vi "XY Drift Test.vi"() -> ()   [LabVIEW 2016]
panel:
  in  "Frame Trigger":i32=500
  out "Frame Number":i32
  out "error out":errorcluster
  in  "Auto XY":bool=TRUE
  out "XY On":bool
  in  "Quit":bool
  in  "Set True":bool
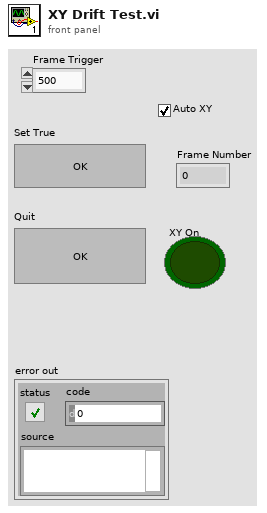
[diagram p1: front panel]
types:
  T1 = typedef "Image Type" = u32
  T2 = typedef "IMAQ Image.ctl" = refnum<image>
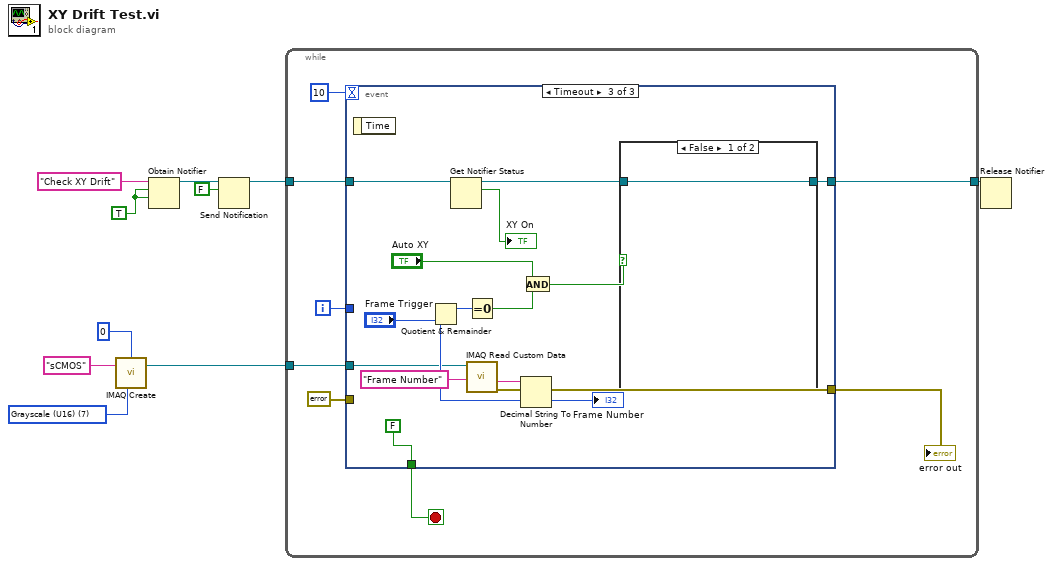
[diagram p0: block diagram]
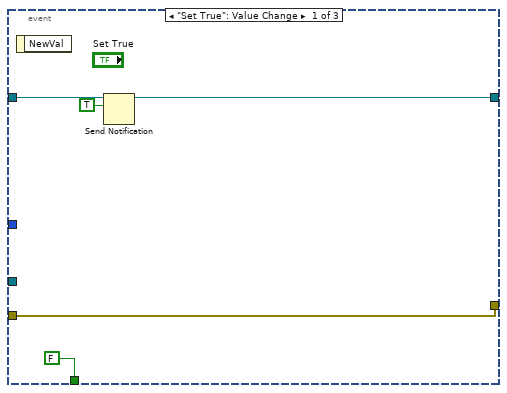
[diagram p2: hidden frame]
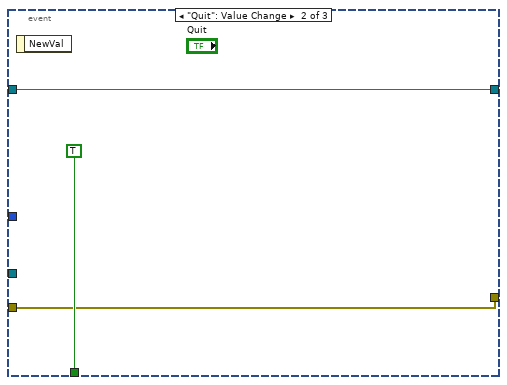
[diagram p3: hidden frame]
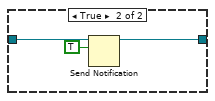
[diagram p4: hidden frame]
diagram:
  w2 = T1 7 items=["Grayscale (U8)", "Grayscale (I16)", "Grayscale (SGL)", "Complex (CSG)", "RGB (U32)", "HSL (U32)", "RGB (U64)", "Grayscale (U16)"] ("Image Type")
  w10 = TRUE ("create if not found? (T)")
  n1 = call "IMAQ Create"("Border Size"=0, "Image Name"="sCMOS" ("name (unnamed)"), "Image Type"=w2) -> ("New Image"=w4:T2)  [unwired: 2 in, 1 out]
  n2 = Obtain Notifier(name (unnamed)="Check XY Drift", notification data type=w10, create if not found? (T)=w10) -> (notifier out=w8:refnum<notifier>)  [unwired: 1 in, 2 out]
  n3 = Send Notification(notification=FALSE, notifier=w8) -> (notifier out=w6:refnum<notifier>)  [unwired: 1 in, 1 out]
  n4 = while {
    tunnel: w6 -> [w17]
    tunnel: [w16] -> w5
    tunnel: w4 -> [w11]
    i -> [w15]
    stop <- w18 stop-if-true
    n5 = event shown="[2] Timeout" {
      selector: _ -> [_ _ _]
      dyn-events: _ -> [_ _ _]
      timeout: 10 -> [_ _ _]
      tunnel: [FALSE ("notification") TRUE ("notification") FALSE ("notification")] -> w18
      tunnel: w17 -> [w22 w26 w40]
      tunnel: [w21 w26 w36] -> w16
      tunnel: w15 -> [_ _ _]
      tunnel: [w19 w24 w31] -> w13
      tunnel: errorcluster {"status"=FALSE, "code"=0, "source"=""} ("error in (no error)") -> [w19 w24 _]
      tunnel: w11 -> [_ _ w29]
      event "Set True": Value Change {
        n6 = event-data() -> ()  [unwired: 1 in, 1 out]
        n7 = Send Notification(notification=TRUE, notifier=w22) -> (notifier out=w21:refnum<notifier>)  [unwired: 1 in, 1 out]
      }
      event "Quit": Value Change {
        n8 = event-data() -> ()  [unwired: 1 in, 1 out]
      }
      event Timeout {
        n9 = event-data() -> ()  [unwired: 1 in, 1 out]
        n10 = Get Notifier Status(notifier=w40) -> (notifier out=w37:refnum<notifier>, current notification=→"XY On":bool)  [unwired: 1 in, 3 out]
        n11 = call "IMAQ Read Custom Data"("Key"="Frame Number", "Image"=w29) -> ("error out"=w31:errorcluster, "Custom Data Out"=w30:string)  [unwired: 7 in, 1 out]
        n12 = Decimal String To Number(string=w30) -> (number=w32:i32)  [unwired: 2 in, 1 out]
        "Frame Number" <- w32
        n13 = Quotient & Remainder(x=w32, y="Frame Trigger") -> (x-y*floor(x/y)=w38:i32)  [unwired: 1 out]
        n14 = Equal To 0?(x=w38) -> (x = 0?=w34:bool)
        n15 = And(x="Auto XY", y=w34) -> (x .and. y?=w35:bool)
        n16 = case shown="False" w35 {
          tunnel: w37 -> [w42 w44]
          tunnel: [w42 w43] -> w36
          frame False {
          }
          frame True {
            n17 = Send Notification(notification=TRUE, notifier=w44) -> (notifier out=w43:refnum<notifier>)  [unwired: 1 in, 1 out]
          }
        }
      }
    }
    "error out" <- w13
  }
  n18 = Release Notifier(notifier=w5) -> ()  [unwired: 2 in, 3 out]
